vi "Enqueue.vi"(8 "error in (no error)":errorcluster, 10 "Data":variant, 11 "Message":string) -> (0 "error out":errorcluster)   [LabVIEW 2010, in "Error Handler.lvlib"]
uses:
  Error Handler.lvlib
  Q Ref FGV Command Enum.ctl
  Q Message Cluster.ctl
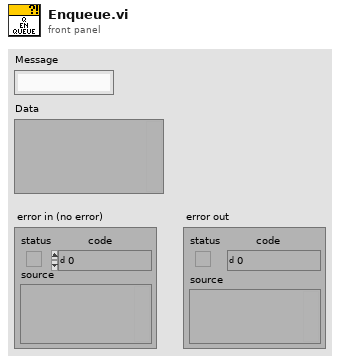
[diagram p1: front panel]
types:
  T1 = typedef "Error Handler.lvlib/Q Message Cluster.ctl" = cluster{"Message":string, "Data":variant}
  T2 = typedef "Error Handler.lvlib/Q Ref FGV Command Enum.ctl" = enum16{"Create Q", "Get Q", "Flush Q", "Release Q"}
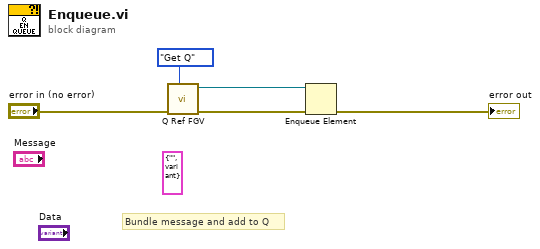
[diagram p0: block diagram]
diagram:
  (unwired) T1 {"Message"="", "Data"=variant} ("element")
  # "Bundle message and add to Q"
  n1 = call "Q Ref FGV.vi"("Command"=Q_Ref_FGV_Command_Enum."Get Q", "error in (no error)"="error in (no error)") -> ("error out"=w1:errorcluster, "Q Ref"=w3:refnum<queue>)  [unwired: 8 in]
  n2 = Enqueue Element(queue=w3, error in (no error)=w1) -> (error out=→"error out":errorcluster)  [unwired: 2 in, 2 out]
